vi "Speed Mode API.vi"(8 "Error in":errorcluster, 10 "String":string, 11 "DVR In":refnum<data-value>) -> (0 "Error out":errorcluster, 2 "This VI":refnum<vi>, 3 "DVR Out":refnum<data-value>)   [LabVIEW 2020, in "Speed Mode.lvclass"]
doc: "To get the refrence of the child function."
uses:
  Speed Mode.lvclass
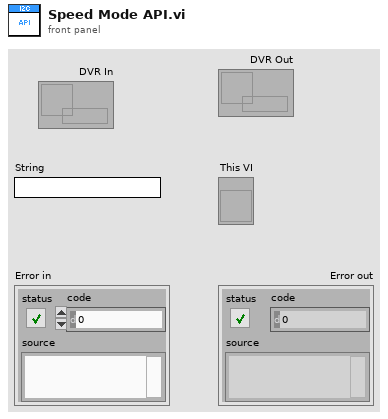
[diagram p1: front panel]
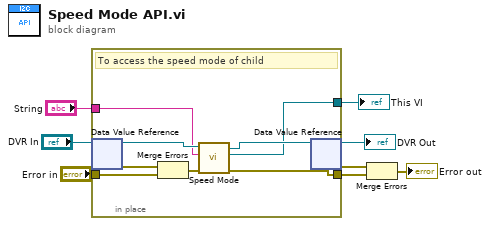
[diagram p0: block diagram]
diagram:
  n1 = in-place {
    in-place-border: "Error in" -> [w12]
    in-place-border: [w11] -> w6
    in-place-border: "String" -> [w10]
    in-place-border: [w9] -> w2
    # "To access the speed mode of child"
    n2 = in-place-dvr #1("DVR In") -> (w16:refnum<class "Speed Mode.lvclass">, w14:errorcluster)
    n3 = Merge Errors(w14, w12) -> (w13:errorcluster)
    n4 = call-dynamic "Speed Mode.vi"("error in (no error)"=w13, "String"=w10, "Speed Mode in"=w16) -> ("error out"=w11:errorcluster, "This VI"=w9:refnum<vi>, "Speed Mode out"=w15:refnum<class "Speed Mode.lvclass">)  [unwired: 6 in]
    n5 = in-place-dvr #1(w15) -> (→"DVR Out":refnum<data-value>, w7:errorcluster)
  }
  "This VI" <- w2
  n6 = Merge Errors(w7, w6) -> (→"Error out":errorcluster)
